vi "Set Single Item.vi"(6 "Child Position":i32=-1, 8 "error in (no error)":errorcluster, 10 "Tree Item In":T1, 11 "Tree in":refnum<class "Tree.lvclass">) -> (0 "error out":errorcluster, 3 "Tree out":refnum<class "Tree.lvclass">)   [LabVIEW 2022 SP3, in "Tree.lvclass"]
uses:
  Tree.lvclass
  Type Def/Tree Item.ctl
  Tree.lvclass/Tree.ctl
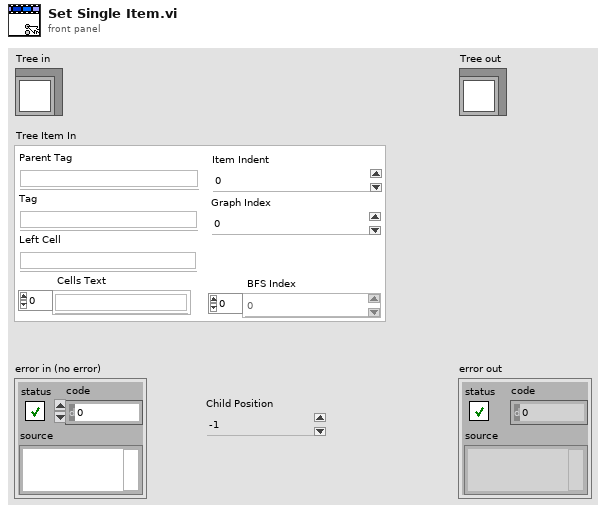
[diagram p1: front panel]
types:
  T1 = typedef "Tree Item.ctl" = cluster{"Parent Tag":string, "Tag":string, "Left Cell":string, "Cells Text":string[], "BFS Index":i32[], "Graph Index":i32, "Item Indent":i32}
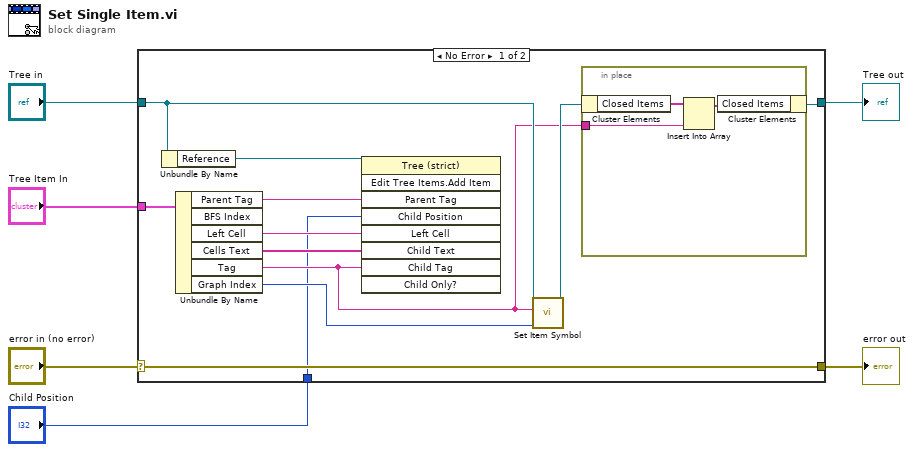
[diagram p0: block diagram]
diagram:
  n1 = case shown="No Error" "error in (no error)" {
    selector: "error in (no error)" -> [w18 w23]
    tunnel: [w18 w23] -> w5
    tunnel: [w9 w22] -> w3
    tunnel: "Tree in" -> [w12 w22]
    tunnel: "Tree Item In" -> [w16 _]
    tunnel: "Child Position" -> [w7 _]
    frame No Error {
      n2 = Unbundle By Name(w12) -> ("Reference"=w17:refnum<vi>)
      n3 = Unbundle By Name(w16) -> ("Parent Tag"=w15:string, "Left Cell"=w14:string, "Cells Text"=w13:string[], "Tag"=w8:string, "Graph Index"=w11:i32)  [unwired: 1 out]
      n4 = invoke class="Tree (strict)" method="Edit Tree Items.Add Item"(reference=w17, "Parent Tag"=w15, "Child Position"=w7, "Left Cell"=w14, "Child Text"=w13, "Child Tag"=w8) -> ()  [unwired: 3 in, 9 out]
      n5 = call "Set Item Symbol.vi"("Symbol"=w11, "Item"=w8, "Tree in"=w12) -> ("Tree out"=w10:refnum<class "Tree.lvclass">)  [unwired: 8 in]
      n6 = in-place {
        in-place-border: w8 -> [w19]
        n7 = in-place-cluster #1(w10) -> ("Closed Items"=w21:string[])
        n8 = Insert Into Array(array=w21, new element=w19) -> (w20:string[])  [unwired: 1 in]
        n9 = in-place-cluster #1("Closed Items"=w20) -> (w9:refnum<class "Tree.lvclass">)
      }
    }
    frame Error {
    }
  }
  "error out" <- w5
  "Tree out" <- w3
